vi "Entry Initialize (User).vi"(8 "error in":errorcluster, 11 "Node in":refnum<class "BLS Chiller Template.lvclass">) -> (0 "error out":errorcluster, 3 "Node out":refnum<class "BLS Chiller Template.lvclass">)   [LabVIEW 2023, in "BLS Chiller Template.lvlib" / "BLS Chiller Template.lvclass"]
uses:
  BLS Chiller Template.lvclass
  BLS Chiller Template.lvclass/BLS Chiller Template.ctl
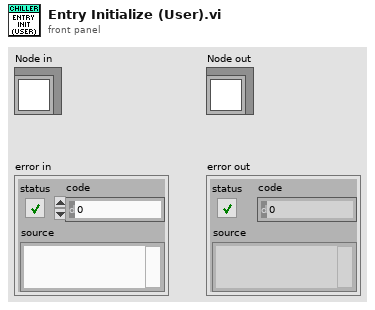
[diagram p1: front panel]
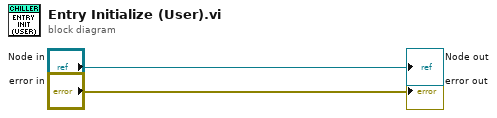
[diagram p0: block diagram]
diagram:
  "Node out" <- "Node in"
  "error out" <- "error in"
